vi "IZMaxSpeed.vi"(2 "ZSpeed":dbl=250.0, 3 "PRIORLib.IZIn":refnum<k7>) -> (0 "error out":errorcluster, 1 "PRIORLib.IZOut":refnum<k7>)   [LabVIEW 2011]
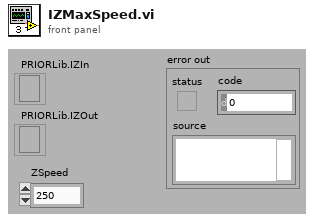
[diagram p1: front panel]
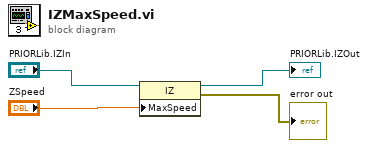
[diagram p0: block diagram]
diagram:
  n1 = property class="IZ"(reference="PRIORLib.IZIn", "MaxSpeed"="ZSpeed") -> (reference out=→"PRIORLib.IZOut":refnum<k7>, error out=→"error out":errorcluster)  [unwired: 1 in]
